vi "Cal Formula.vi"(5 "Format":T2 items=["Decimal"=0, "Scientific"=1, "Hexadecimal"=5], 7 "precision (6)":i16, 8 "error in (no error)":errorcluster caption="错误输入（无错误）", 10 "Formula In":string, 11 "Data In":T1) -> (0 "error out":errorcluster caption="错误输出", 2 "Numeric String":string, 3 "Data Out":dbl format="%0.2f")   [LabVIEW 2013, in "Calculator XControl.xctl"]
uses:
  Calculator XControl.xctl
  Controls/Format.ctl
  Core/Data.ctl
  <vilib>/gmath/NI_Gmath.lvlib
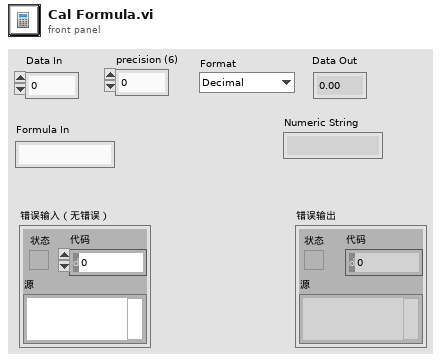
[diagram p1: front panel]
types:
  T1 = typedef "Calculator XControl.xctl/Data.ctl" = dbl
  T2 = typedef "Calculator XControl.xctl/Format.ctl" = u16
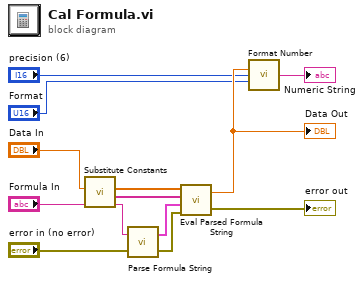
[diagram p0: block diagram]
diagram:
  n1 = call "Substitute Constants.vi"("Formula In"="Formula In", "Data In"="Data In") -> ("Formula Out"=w13:string, "Variables Out"=w12:string[], "Values Out"=w11:dbl[])  [unwired: 7 in]
  n2 = call <vilib>:"Parse Formula String.vi"("error in (no error)"="error in (no error)", "formula"=w13) -> ("error out"=w9:errorcluster, "Parsed Formula"=w10:cluster{"Table":i32[][], "Y Values":dbl[]})
  n3 = call <vilib>:"Eval Parsed Formula String.vi"("error in (no error)"=w9, "Parsed Formula"=w10, "Variables"=w12, "X Values"=w11) -> ("error out"=→"error out":errorcluster, "y value"=w5:dbl)
  "Data Out" <- w5
  n4 = call "Format Number.vi"("Data"=w5, "precision (6)"="precision (6)", "Format"="Format") -> ("Numeric String"=→"Numeric String":string)  [unwired: 12 in]
